vi "Camera_Exposure.vi"(8 "error in":errorcluster, 10 "Action":enum16{"Write", "Read"}(ring), 11 "Exposure (s)":dbl=1000.0 format="%0.2f") -> (0 "error out":errorcluster, 3 "Exposure (s)":dbl=1000.0 format="%0.2f")   [LabVIEW 2025]
doc: "Functional Global Variable:\n- Write the value into the memory \nor\n- Read the value from the memory"
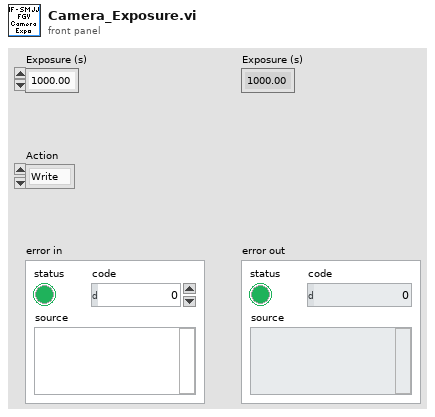
[diagram p1: front panel]
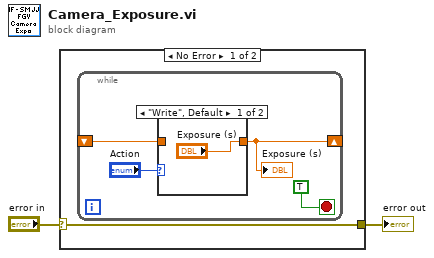
[diagram p0: block diagram]
diagram:
  n1 = case shown="No Error" "error in" {
    selector: "error in" -> [w3 w10]
    tunnel: [w3 w10] -> w1
    frame No Error {
      n2 = while {
        shift-right: [w4] -> _
        shift-left: _ -> [w5]
        stop <- TRUE stop-if-true
        n3 = case shown="\"Write\", Default" "Action" {
          tunnel: w5 -> [_ w9]
          tunnel: ["Exposure (s)" w9] -> w4
          frame "Write", Default {
          }
          frame "Read" {
          }
        }
        "Exposure (s)" <- w4
      }
    }
    frame Error {
    }
  }
  "error out" <- w1
